vi "check_is_moving.vi"(8 "error in (no error)":errorcluster, 11 "XPS control in":refnum<class "XPS.lvclass">) -> (0 "error out":errorcluster, 2 "Numeric":dbl, 3 "XPS control out":refnum<class "XPS.lvclass">)   [LabVIEW 2019, in "XPS.lvlib" / "XPS.lvclass"]
uses:
  XPS.lvclass
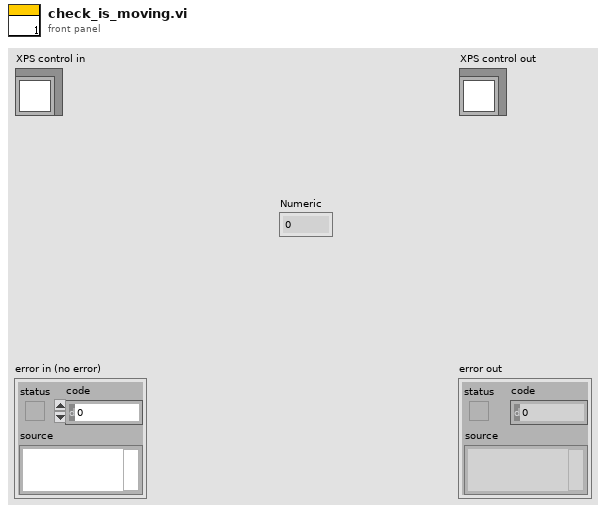
[diagram p1: front panel]
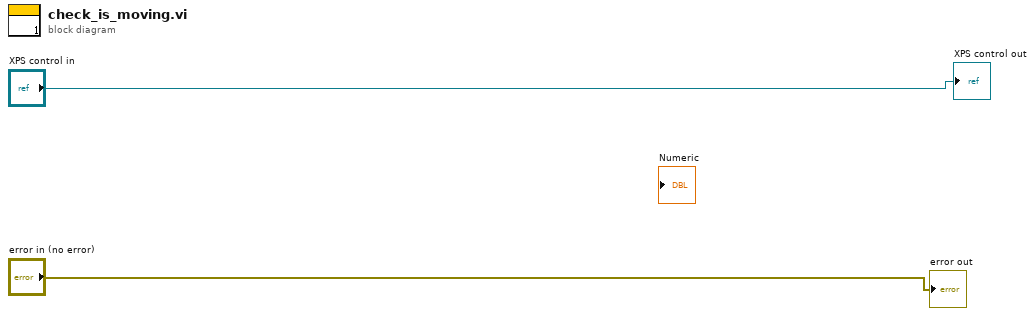
[diagram p0: block diagram]
diagram:
  "error out" <- "error in (no error)"
  "XPS control out" <- "XPS control in"
